vi "createBroadcastFreezeSensorValuesFrame.vi"(0 "HPILC in":refnum<class "HPILC.lvclass">, 5 "WaitForTrigger":bool, 7 "TriggerIRQ":bool, 9 "BroadcastCounter":u8, 11 "error in (no error)":errorcluster) -> (4 "HPILC out":refnum<class "HPILC.lvclass">, 6 "TxFrame":T1 {"Data" format="%02x"}, 15 "error out":errorcluster)   [LabVIEW 2016, in "RTHPILC.lvlib" / "HPILC.lvclass"]
uses:
  HPILC.lvclass
  Common_RT_Modbus/DataTypes/TxFrame.ctl
  Common_RT_Modbus/DynamicFrameBuilder/DynamicFrameBuilder.lvclass
  HPILC.lvclass/HPILC.ctl
  Common_RT_Modbus/RTModbus.lvlib
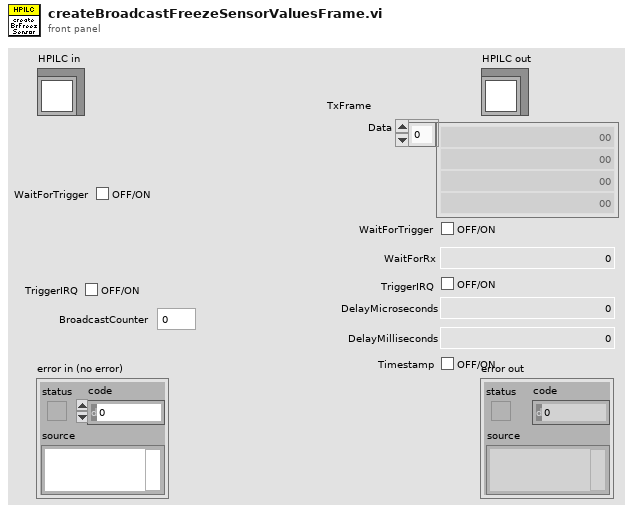
[diagram p1: front panel]
types:
  T1 = typedef "RTModbus.lvlib/TxFrame.ctl" = cluster{"Data":u8[], "WaitForTrigger":bool, "WaitForRx":u16, "TriggerIRQ":bool, "DelayMicroseconds":u16, "DelayMilliseconds":u16, "Timestamp":bool}
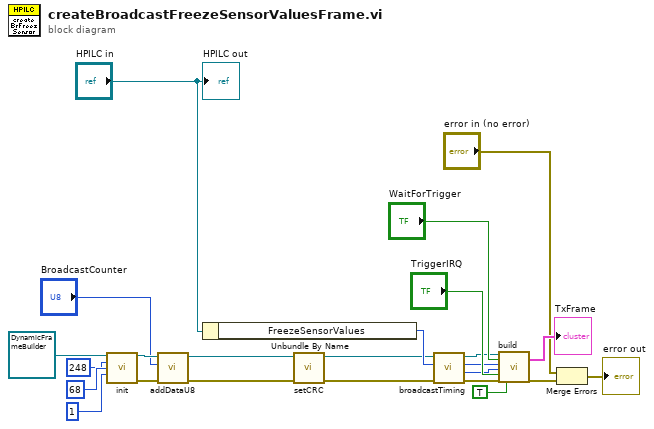
[diagram p0: block diagram]
diagram:
  n1 = call "init.vi"("DynamicFrameBuilder in"=refnum<class "DynamicFrameBuilder.lvclass"> refnum ("RTModbus.lvlib:DynamicFrameBuilder.lvclass"), "Address"=u8 248, "Function"=u8 68, "DataSize"=1) -> ("DynamicFrameBuilder out"=w14:refnum<class "DynamicFrameBuilder.lvclass">, "error out"=w12:errorcluster)  [unwired: 10 in]
  n2 = call "addDataU8.vi"("error in (no error)"=w12, "Data"="BroadcastCounter", "DynamicFrameBuilder in"=w14) -> ("error out"=w11:errorcluster, "DynamicFrameBuilder out"=w10:refnum<class "DynamicFrameBuilder.lvclass">)  [unwired: 7 in]
  n3 = Unbundle By Name("HPILC in") -> ("FreezeSensorValues"=w8:u32)
  n4 = call "setCRC.vi"("error in (no error)"=w11, "DynamicFrameBuilder in"=w10) -> ("error out"=w6:errorcluster, "DynamicFrameBuilder out"=w7:refnum<class "DynamicFrameBuilder.lvclass">)  [unwired: 8 in]
  n5 = call "broadcastTiming.vi"("error in (no error)"=w6, "Latency in"=w8, "DynamicFrameBuilder in"=w7) -> ("error out"=w4:errorcluster, "WaitForRxTimeout"=w2:u16, "Latency out"=w3:u32, "DynamicFrameBuilder out"=w5:refnum<class "DynamicFrameBuilder.lvclass">)  [unwired: 5 in]
  n6 = call "build.vi"("DynamicFrameBuilder in"=w5, "WaitForTrigger"="WaitForTrigger", "Latency"=w3, "WaitForRxTimeout"=w2, "TriggerIRQ"="TriggerIRQ", "error in (no error)"=w4, "Timestamp"=TRUE) -> ("TxFrame"=→"TxFrame":T1, "error out"=w20:errorcluster)  [unwired: 10 in, 1 out]
  n7 = Merge Errors("error in (no error)", w20) -> (→"error out":errorcluster)
  "HPILC out" <- "HPILC in"
